vi "Update GPU UI Components.vi"(8 "error in (no error)":errorcluster, 10 "GPU UI metrics":T1, 11 "Application Manager in":refnum<class "Application Manager.lvclass">) -> (0 "error out":errorcluster, 3 "Application Manager out":refnum<class "Application Manager.lvclass">)   [LabVIEW 2020, in "Application Manager.lvlib" / "Application Manager.lvclass"]
uses:
  Application Manager.lvclass
  Simple UI/Simple UI/GPU Batch Results.ctl
  Application Manager.lvclass/Application Manager.ctl
  Simple UI/Simple UI/Simple UI.lvclass
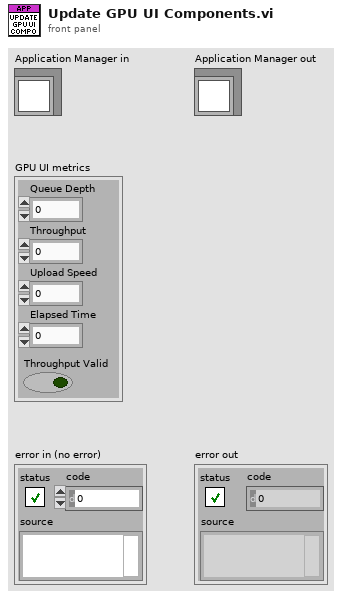
[diagram p1: front panel]
types:
  T1 = typedef "Simple UI.lvlib/Simple UI.lvclass/GPU Batch Results.ctl" = cluster{"Queue Depth":dbl, "Throughput":dbl, "Upload Speed":dbl, "Elapsed Time":dbl, "Throughput Valid":bool}
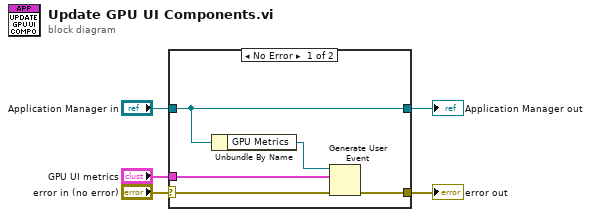
[diagram p0: block diagram]
diagram:
  n1 = case shown="No Error" "error in (no error)" {
    selector: "error in (no error)" -> [w8 w12]
    tunnel: [w7 w12] -> w4
    tunnel: [w10 w11] -> w2
    tunnel: "Application Manager in" -> [w10 w11]
    tunnel: "GPU UI metrics" -> [w6 _]
    frame No Error {
      n2 = Unbundle By Name(w10) -> ("GPU Metrics"=w9:refnum<user-event>)
      n3 = Generate User Event(user event=w9, event data cluster=w6, error in=w8) -> (error out=w7:errorcluster)  [unwired: 1 in, 1 out]
    }
    frame Error {
    }
  }
  "error out" <- w4
  "Application Manager out" <- w2
